vi "GetSNCurrentStatus.vi"(0 "class data in":refnum<class "CMESAPI.lvclass">, 5 "serialNumber":string, 11 "error in (no error)":errorcluster) -> (4 "class data out":refnum<class "CMESAPI.lvclass">, 6 "GetSNCurrentStatus":string, 8 "resulting string":string, 15 "error out":errorcluster)   [LabVIEW 2020, in "Salcomp-MES.lvlib" / "CMESAPI.lvclass"]
uses:
  CMESAPI.lvclass
  CMESAPI.lvclass/CMESAPI.ctl
  E:/Git/Libraries/develop/CME-API/CMESAPI_Fw4.0_1.9.2/CMESAPI.dll
  CMESAPI_Fw4.0_1.9.2/CMESAPI.dll
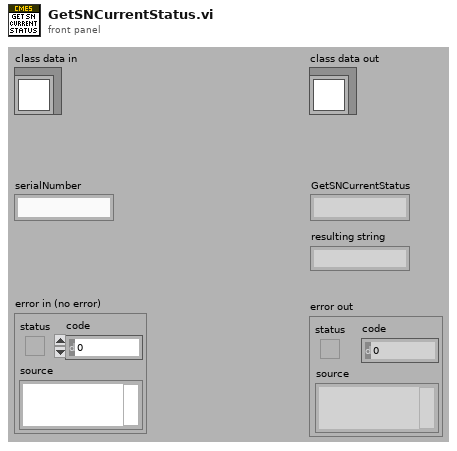
[diagram p1: front panel]
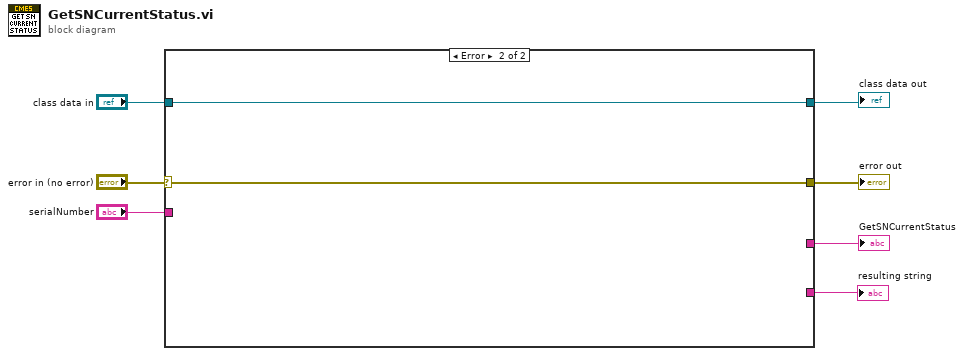
[diagram p0: block diagram]
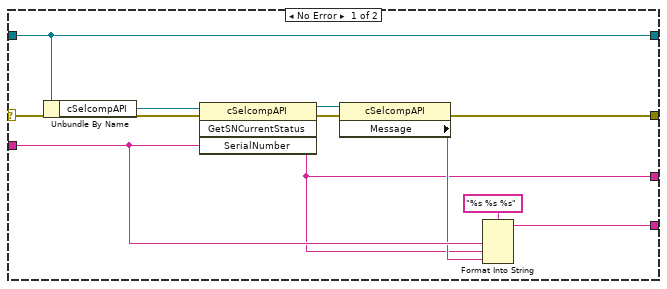
[diagram p2: hidden frame]
diagram:
  n1 = case shown="Error" "error in (no error)" {
    selector: "error in (no error)" -> [w16 w20]
    tunnel: [w13 w20] -> w6
    tunnel: "class data in" -> [w18 w19]
    tunnel: [w18 w19] -> w4
    tunnel: "serialNumber" -> [w11 _]
    tunnel: [w9 _] -> w2
    tunnel: [w8 _] -> w1
    frame No Error {
      n2 = Unbundle By Name(w18) -> ("cSelcompAPI"=w17:refnum<k24>)
      n3 = invoke on="Invoke Node" class="cSelcompAPI" method="GetSNCurrentStatus"(reference=w17, error in=w16, "SerialNumber"=w11) -> (reference out=w12:refnum<k24>, error out=w14:errorcluster, "GetSNCurrentStatus"=w9:string)  [unwired: 1 in, 1 out]
      n4 = property class="cSelcompAPI"(reference=w12, error in=w14) -> (error out=w13:errorcluster, "Message"=w10:string)  [unwired: 1 out]
      n5 = Format Into String(format string="%s %s %s", w11, w9, w10) -> (resulting string=w8:string)  [unwired: 2 in, 1 out]
    }
    frame Error {
    }
  }
  "error out" <- w6
  "class data out" <- w4
  "GetSNCurrentStatus" <- w2
  "resulting string" <- w1
